vi "Supported Smart Syntax Representation.vi"(0 "Message Popup in":refnum<class "Message Popup.lvclass">, 11 "error in (no error)":errorcluster) -> (4 "Message Popup out":refnum<class "Message Popup.lvclass">, 6 "Smart Syntax Representation List":string[](array[string]), 15 "error out":errorcluster)   [LabVIEW 2016, in "Message Popup.lvclass"]
uses:
  Message Popup.lvclass
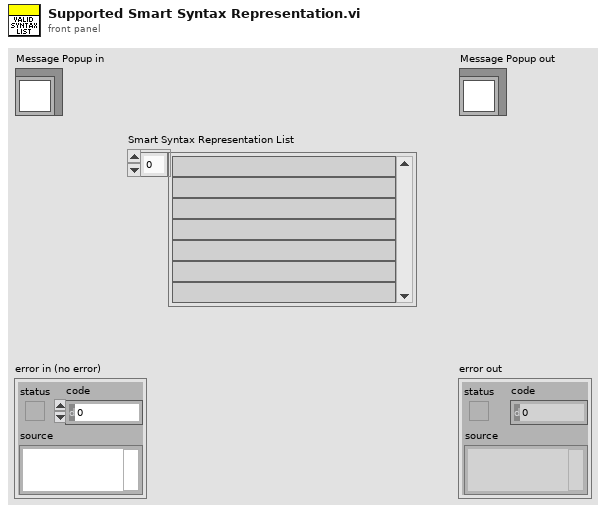
[diagram p1: front panel]
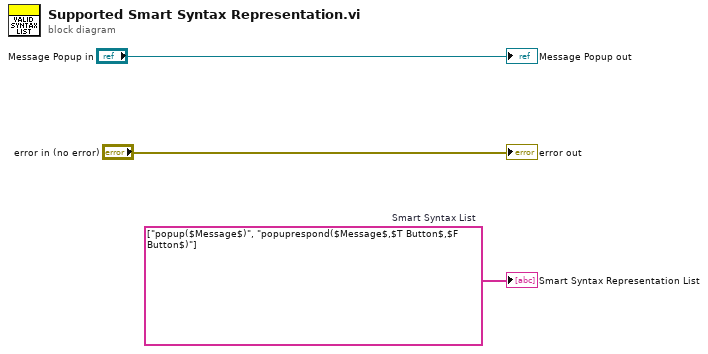
[diagram p0: block diagram]
diagram:
  w1 = string[] ["popup($Message$)", "popuprespond($Message$,$T Button$,$F Button$)"]  # Smart Syntax List
  "error out" <- "error in (no error)"
  "Message Popup out" <- "Message Popup in"
  "Smart Syntax Representation List" <- w1
